vi "Send Commands.vi"(8 "error in":errorcluster, 10 "Set Temp":dbl, 11 "Network Stream in":refnum<class "Network Stream.lvclass">) -> (0 "error out":errorcluster, 3 "Network Stream out":refnum<class "Network Stream.lvclass">)   [LabVIEW 2019, in "Network Stream.lvlib" / "Network Stream.lvclass"]
uses:
  Network Stream.lvclass
  Network Stream.lvclass/Network Stream.ctl
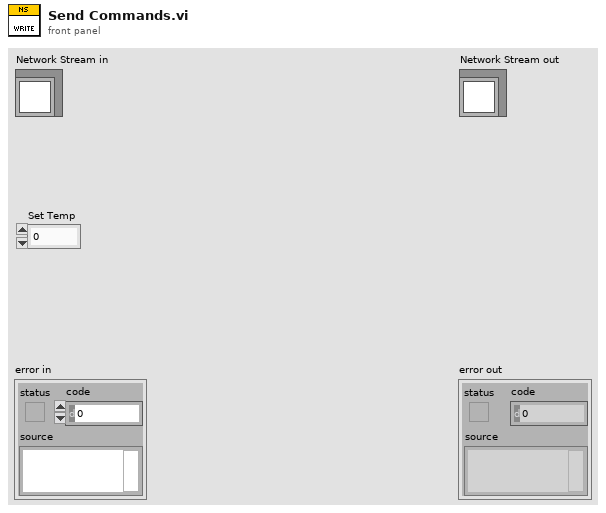
[diagram p1: front panel]
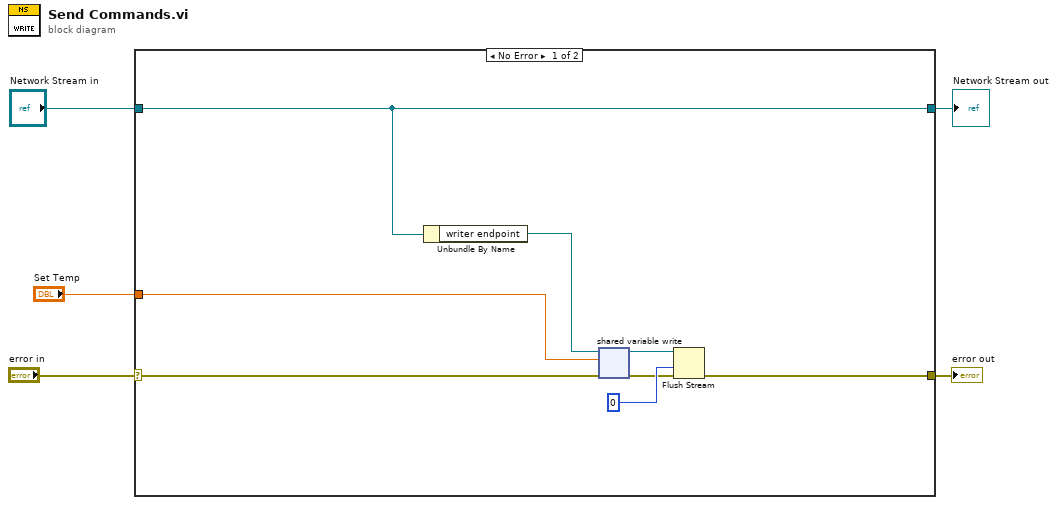
[diagram p0: block diagram]
diagram:
  n1 = case shown="No Error" "error in" {
    selector: "error in" -> [w10 w15]
    tunnel: [w9 w15] -> w4
    tunnel: [w8 w14] -> w2
    tunnel: "Network Stream in" -> [w8 w14]
    tunnel: "Set Temp" -> [w6 _]
    frame No Error {
      n2 = Unbundle By Name(w8) -> ("writer endpoint"=w7:refnum<k21>)
      n3 = shared-variable-write(w7, w10, w6) -> (w12:refnum<k21>, w11:errorcluster)  [unwired: 1 in, 1 out]
      n4 = Flush Stream(8:w11, 9:0 ("timeout in ms (-1)"), 11:w12) -> (0:w9:errorcluster)  [unwired: 1 in, 2 out]
    }
    frame Error {
    }
  }
  "error out" <- w4
  "Network Stream out" <- w2
